vi "Read.vi"(11 "TaskEnQrValue in":refnum<class "TaskEnQrValue.lvclass">) -> (2 "EnQr":refnum<class "Message Enqueuer.lvclass">)   [LabVIEW 2020, in "Volatus.lvlib" / "TaskEnQrValue.lvclass"]
uses:
  TaskEnQrValue.lvclass
  TaskEnQrValue.lvclass/TaskEnQrValue.ctl
  <vilib>/ActorFramework/Message Enqueuer/Message Enqueuer.lvclass
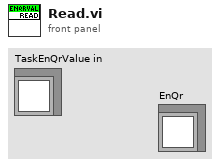
[diagram p1: front panel]
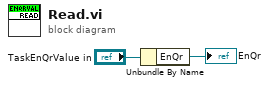
[diagram p0: block diagram]
diagram:
  n1 = Unbundle By Name("TaskEnQrValue in") -> ("EnQr"=→"EnQr":refnum<class "Message Enqueuer.lvclass">)
